vi "IC_Sink_Grab_Picture.vi"(0 "ICImagingControl In":refnum<k7>, 1 "Error In (no error)":errorcluster) -> (2 "ICImagingControl Out":refnum<k7>, 3 "Picture Out":picture, 4 "SampleStartTime":dbl, 5 "Error Out":errorcluster)   [LabVIEW 2020]
doc: "This VI grabs an image from the live video stream and returns a picture. It uses a previously by IC_CreateFrameHandlerSink created sink. It must be used, if frame filters are in use by IC Imaging Control."
uses:
  <vilib>/picture/picture.llb/Draw 8-Bit Pixmap.vi
  <vilib>/picture/picture.llb/Draw True-Color Pixmap.vi
  <userlib>/IC LabVIEW Extension 2.dll
panel:
  in  "Case Constant\n(See Context Help)":bool=TRUE
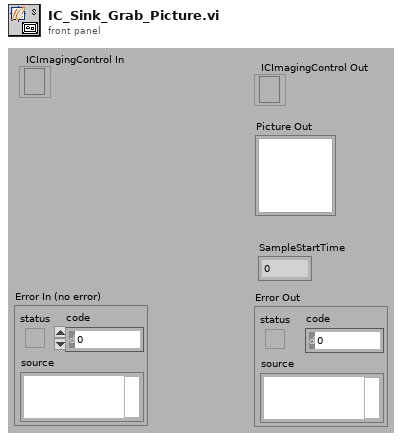
[diagram p1: front panel]
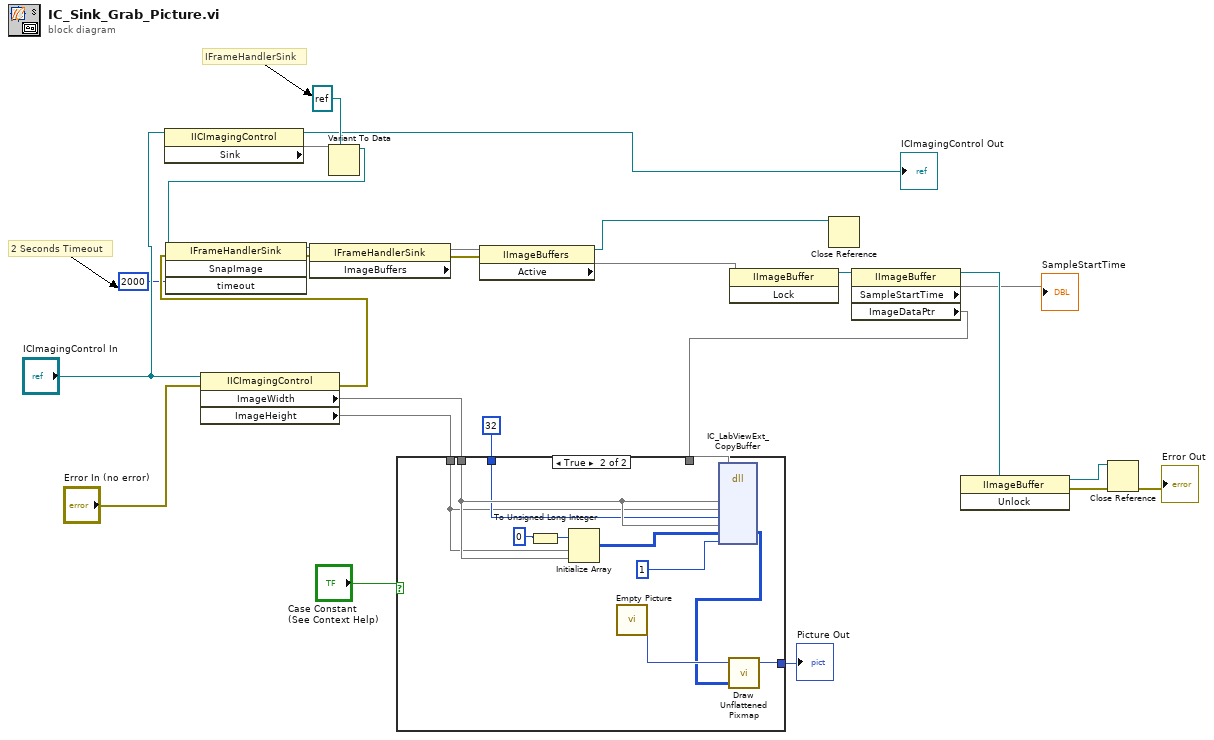
[diagram p0: block diagram]
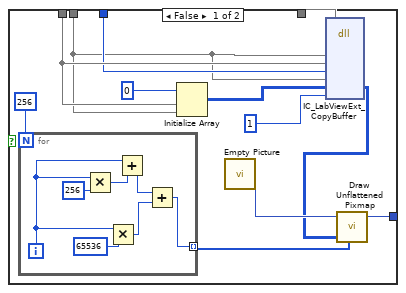
[diagram p2: hidden frame]
diagram:
  # "2 Seconds Timeout"
  # "IFrameHandlerSink"
  n1 = property class="IICImagingControl"(reference="ICImagingControl In") -> (reference out=→"ICImagingControl Out":refnum<k7>, "Sink"=w9)  [unwired: 1 in, 1 out]
  n2 = property class="IICImagingControl"(reference="ICImagingControl In", error in="Error In (no error)") -> (error out=w22:errorcluster, "ImageWidth"=w25, "ImageHeight"=w26)  [unwired: 1 out]
  n3 = Variant To Data(type=refnum<k7> refnum ("ICImagingControl3.IFrameHandlerSink"), Variant=w9) -> (data=w7:refnum<k7>)  [unwired: 1 in, 1 out]
  n4 = invoke class="IFrameHandlerSink" method="SnapImage"(reference=w7, error in=w22, "timeout"=2000) -> (reference out=w21:refnum<k7>, error out=w20:errorcluster)  [unwired: 1 in, 2 out]
  n5 = property class="IFrameHandlerSink"(reference=w21, error in=w20) -> (error out=w19:errorcluster, "ImageBuffers"=w18)  [unwired: 1 out]
  n6 = property class="IImageBuffers"(reference=w18, error in=w19) -> (reference out=w5:refnum<k7>, "Active"=w4)  [unwired: 1 out]
  n7 = invoke class="IImageBuffer" method="Lock"(reference=w4) -> (reference out=w11:refnum<k7>)  [unwired: 2 in, 2 out]
  n8 = Close Reference(reference=w5) -> ()  [unwired: 1 in, 1 out]
  n9 = property class="IImageBuffer"(reference=w11) -> (reference out=w17:refnum<k7>, "SampleStartTime"=→"SampleStartTime", "ImageDataPtr"=w12)  [unwired: 1 in, 1 out]
  n10 = case shown="True" "Case Constant\n(See Context Help)" {
    tunnel: w26 -> [w33 w47]
    tunnel: w25 -> [w31 w54]
    tunnel: 32 ("ImageBitsPerPixel") -> [w32 w50]
    tunnel: [w36 w56] -> w24
    tunnel: w12 -> [w27 w46]
    frame False {
      n11 = for {
        N: 256 -> [_]
        tunnel: [w39] -> w34 mode=indexing
        i -> [w40]
        n12 = Multiply(x=w40, y=256) -> (x*y=w43:i32)
        n13 = Multiply(x=w40, y=65536) -> (x*y=w45:i32)
        n14 = Add(x=w40, y=w43) -> (x+y=w41:i32)
        n15 = Add(x=w41, y=w45) -> (x+y=w39:i32)
      }
      n16 = Initialize Array(u8 0, w33, w31) -> (w30:u8[][])
      n17 = call "Empty Picture"() -> ("empty picture"=w38:picture)
      n18 = dll-call lib="C:/Programme/National Instruments/LabVIEW 7.0/user.lib/IC LabVIEW Extension.dll" fn="IC_LabViewExt_CopyBuffer"("data"=w27, "width"=w31, "height"=w33, "bpp"=w32, "imaq_width"=w31, "imaq_ptr"=w30, "bFlip"=1) -> ("imaq_ptr"=w28:u8[][])  [unwired: 10 in, 2 out]
      n19 = call-poly <vilib>:"Draw Unflattened Pixmap.vi"("picture"=w38, "data"=w28, "color table"=w34) -> ("new picture"=w36:picture)  [unwired: 6 in]
    }
    frame True {
      n20 = To Unsigned Long Integer(number=u8 0) -> (unsigned 32bit integer=w48:u32)
      n21 = Initialize Array(w48, w47, w54) -> (w53:u32[][])
      n22 = call "Empty Picture"() -> ("empty picture"=w55:picture)
      n23 = dll-call lib="C:/Programme/National Instruments/LabVIEW 7.0/user.lib/IC LabVIEW Extension.dll" fn="IC_LabViewExt_CopyBuffer"("data"=w46, "width"=w54, "height"=w47, "bpp"=w50, "imaq_width"=w54, "imaq_ptr"=w53, "bFlip"=1) -> ("imaq_ptr"=w51:u32[][])  [unwired: 10 in, 2 out]
      n24 = call-poly <vilib>:"Draw Unflattened Pixmap.vi"("picture"=w55, "data (RGB format)"=w51) -> ("new picture"=w56:picture)  [unwired: 7 in]
    }
  }
  "Picture Out" <- w24
  n25 = invoke class="IImageBuffer" method="Unlock"(reference=w17) -> (reference out=w13:refnum<k7>, error out=w15:errorcluster)  [unwired: 2 in, 1 out]
  n26 = Close Reference(reference=w13, error in (no error)=w15) -> (error out=→"Error Out":errorcluster)
